vi "PCO_Binning.vi"(8 "error in":errorcluster, 10 "Binning":u16(ring)=2 items=["1x1"=1, "2x2"=2, "4x4"=4, "8x8"=8], 11 "Data":u16[][](array[numeric])) -> (0 "error out":errorcluster, 3 "Data bin":dbl[][](array[numeric]))   [LabVIEW 2024]
uses:
  <vilib>/Analysis/NI_AALBase.lvlib
  <vilib>/Analysis/baseanly.llb/Mean (DBL).vi
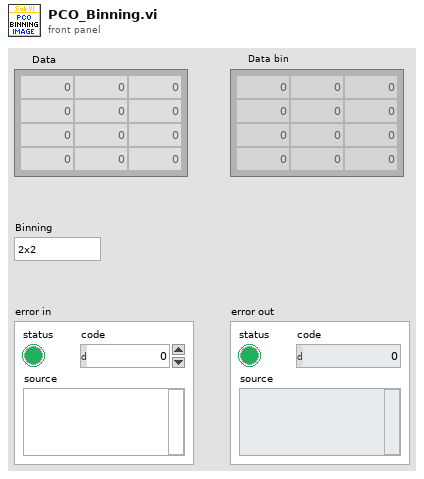
[diagram p1: front panel]
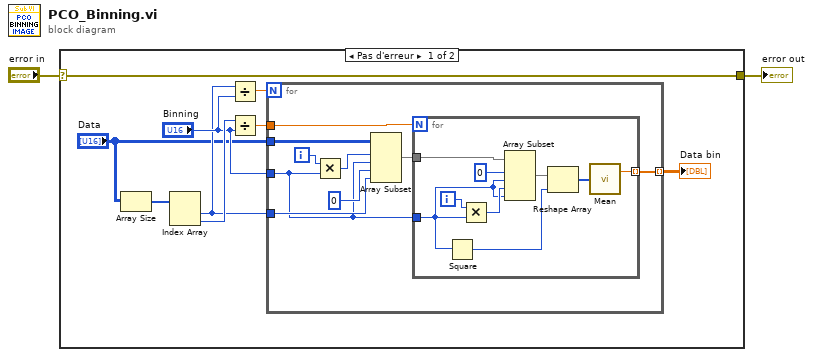
[diagram p0: block diagram]
diagram:
  n1 = case shown="Pas d'erreur" "error in" {
    selector: "error in" -> [w11 w30]
    tunnel: [w11 w30] -> w1
    frame No Error {
      n2 = Array Size(array="Data") -> (size(s)=w10:i32[])
      n3 = Index Array(array=w10) -> (element #1=w6:i32, element #2=w9:i32)  [unwired: 2 in]
      n4 = Divide(x=w6, y="Binning") -> (x/y=w8:dbl)
      n5 = Divide(x=w9, y="Binning") -> (x/y=w5:dbl)
      n6 = for {
        N: w8 -> [_]
        tunnel: "Binning" -> [w14]
        tunnel: "Data" -> [w19]
        tunnel: w6 -> [w16]
        tunnel: w5 -> [w15]
        tunnel: [w12] -> w4 mode=indexing
        i -> [w20]
        n7 = Multiply(x=w20, y=w14) -> (x*y=w18:i32)
        n8 = Array Subset(array=w19, index (row)=w18, length (row)=w14, index (col)=0 ("indice"), length (col)=w16) -> (w13:u16[][])
        n9 = for {
          N: w15 -> [_]
          tunnel: w14 -> [w24]
          tunnel: w13 -> [w28]
          tunnel: [w21] -> w12 mode=indexing
          i -> [w29]
          n10 = Square(x=w24) -> (x^2=w23:u16)
          n11 = Multiply(x=w29, y=w24) -> (x*y=w26:i32)
          n12 = Array Subset(array=w28, index (row)=0 ("indice"), length (row)=w24, index (col)=w26, length (col)=w24) -> (w25:u16[][])
          n13 = Reshape Array(w25, w23) -> (w22:u16[])
          n14 = call-poly <vilib>:"Mean.vi"("X"=w22) -> ("mean"=w21:dbl)  [unwired: 1 out]
        }
      }
      "Data bin" <- w4
    }
    frame Error {
    }
  }
  "error out" <- w1
